vi "get_mux.vi"(8 "error in (no error)":errorcluster, 10 "Channel":string, 11 "Agilent 34980A in":refnum<class "Agilent 34980A.lvclass">) -> (0 "error out":errorcluster, 2 "value":string, 3 "Agilent 34980A out":refnum<class "Agilent 34980A.lvclass">)   [LabVIEW 2018, in "Agilent 34980A.lvclass"]
doc: "Agilent:\nread the voltage of a channel from the MUX slot"
uses:
  Agilent 34980A.lvclass
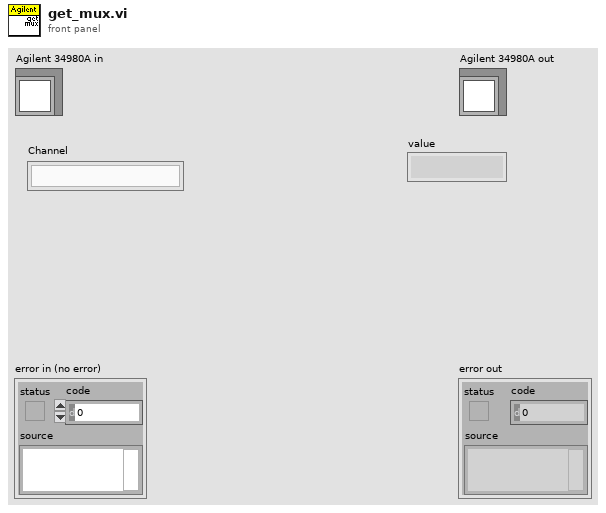
[diagram p1: front panel]
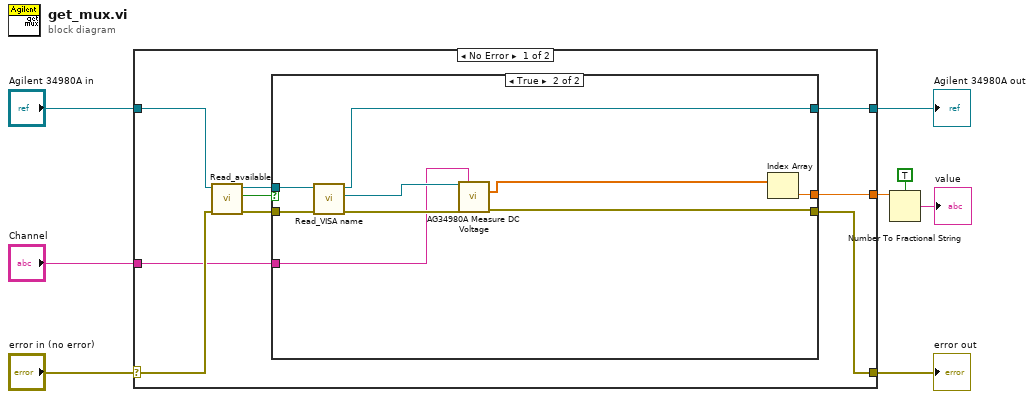
[diagram p0: block diagram]
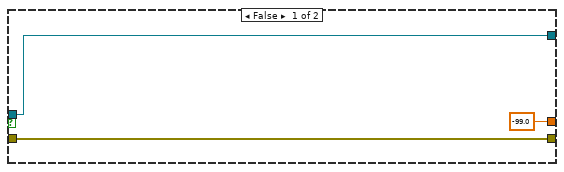
[diagram p2: hidden frame]
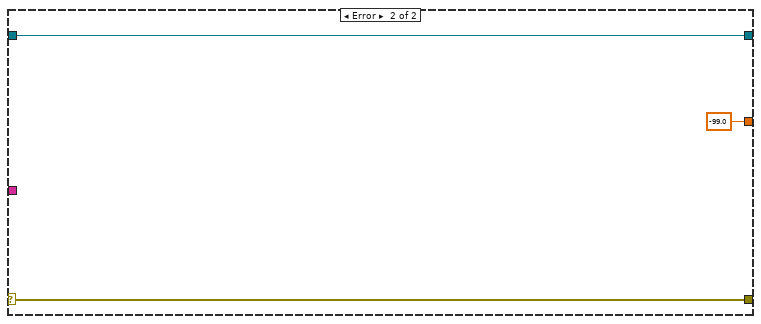
[diagram p3: hidden frame]
diagram:
  n1 = case shown="No Error" "error in (no error)" {
    selector: "error in (no error)" -> [w16 w32]
    tunnel: [w11 w32] -> w7
    tunnel: [w13 w31] -> w5
    tunnel: "Agilent 34980A in" -> [w17 w31]
    tunnel: "Channel" -> [w10 _]
    tunnel: [w9 -99.0] -> w3
    frame No Error {
      n2 = call-dynamic "Read_available.vi"("error in (no error)"=w16, "instrument in"=w17) -> ("error out"=w12:errorcluster, "available?"=w15:bool, "instrument out"=w14:refnum<class "Agilent 34980A.lvclass">)  [unwired: 7 in]
      n3 = case shown="True" w15 {
        tunnel: w14 -> [w20 w29]
        tunnel: [w20 w28] -> w13
        tunnel: w12 -> [w19 w27]
        tunnel: [w19 w22] -> w11
        tunnel: w10 -> [_ w23]
        tunnel: [-99.0 w26] -> w9
        frame False {
        }
        frame True {
          n4 = call-dynamic "Read_VISA name.vi"("error in (no error)"=w27, "instrument in"=w29) -> ("error out"=w25:errorcluster, "VISA resource name"=w24:refnum<visa-resource-name>, "instrument out"=w28:refnum<class "Agilent 34980A.lvclass">)  [unwired: 7 in]
          n5 = call "AG34980A Measure DC Voltage.vi"("VISA resource name"=w24, "Channel List(empty)"=w23, "error in (no error)"=w25) -> ("Output Array"=w21:dbl[], "error out"=w22:errorcluster)  [unwired: 10 in, 1 out]
          n6 = Index Array(array=w21) -> (element=w26:dbl)  [unwired: 1 in]
        }
      }
    }
    frame Error {
    }
  }
  "error out" <- w7
  "Agilent 34980A out" <- w5
  n7 = Number To Fractional String(use system decimal point (T)=TRUE, number=w3) -> (F-format string=→"value":string)  [unwired: 2 in]
